vi "Initialize.vi"(8 "error in (no error)":errorcluster, 11 "Component UI in":refnum<class "Core Configuration UI.lvclass">) -> (0 "error out":errorcluster, 3 "Component UI out":refnum<class "Core Configuration UI.lvclass">)   [LabVIEW 2017, in "DSF Core.lvlib" / "Core Configuration UI.lvclass"]
uses:
  Core Configuration UI.lvclass
  C:/Git/DSF/Core/Classes/Component User Interface/Component User Interface.lvclass
  Channel/Core Channel User Interface.lvclass
  C:/Git/DSF/Core/Classes/User Interface/User Interface.lvclass
  Group/Core Group User Interface.lvclass
  Plugin/Core Plugin User Interface.lvclass
  Thread/Core Thread User Interface.lvclass
  Transfer/Core Transfer User Interface.lvclass
  Component User Interface/Component User Interface.lvclass
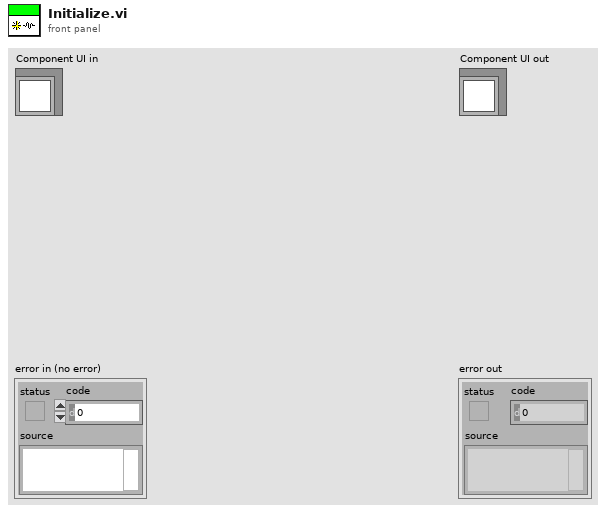
[diagram p1: front panel]
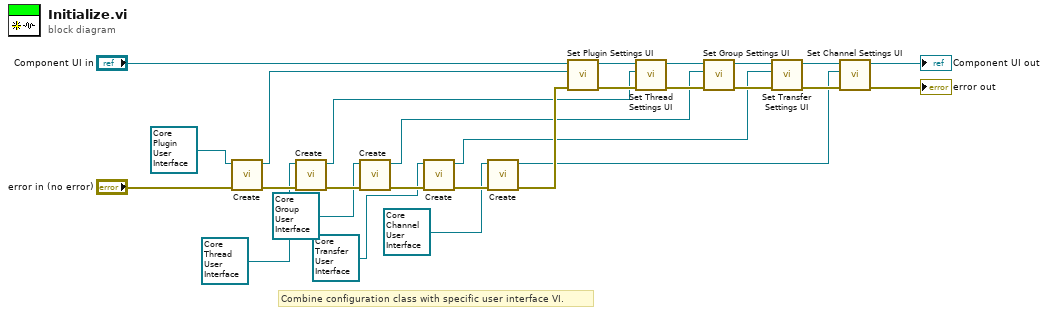
[diagram p0: block diagram]
diagram:
  # "Combine configuration class with specific user interface VI."
  n1 = call-dynamic "Create.vi"("error in (no error)"="error in (no error)", "Core Plugin User Interface in"=refnum<class "Core Plugin User Interface.lvclass"> refnum ("DSF Core.lvlib:Core Plugin User Interface.lvclass")) -> ("error out"=w5:errorcluster, "Core Plugin User Interface out"=w12:refnum<class "Core Plugin User Interface.lvclass">)  [unwired: 8 in]
  n2 = call-dynamic "Create.vi"("error in (no error)"=w5, "Core Thread User Interface in"=refnum<class "Core Thread User Interface.lvclass"> refnum ("DSF Core.lvlib:Core Thread User Interface.lvclass")) -> ("error out"=w27:errorcluster, "Core Thread User Interface out"=w11:refnum<class "Core Thread User Interface.lvclass">)  [unwired: 8 in]
  n3 = call-dynamic "Create.vi"("error in (no error)"=w27, "Core Group User Interface in"=refnum<class "Core Group User Interface.lvclass"> refnum ("DSF Core.lvlib:Core Group User Interface.lvclass")) -> ("error out"=w26:errorcluster, "Core Group User Interface out"=w10:refnum<class "Core Group User Interface.lvclass">)  [unwired: 8 in]
  n4 = call-dynamic "Create.vi"("error in (no error)"=w26, "Core Transfer User Interface in"=refnum<class "Core Transfer User Interface.lvclass"> refnum ("DSF Core.lvlib:Core Transfer User Interface.lvclass")) -> ("error out"=w25:errorcluster, "Core Transfer User Interface out"=w9:refnum<class "Core Transfer User Interface.lvclass">)  [unwired: 8 in]
  n5 = call-dynamic "Create.vi"("error in (no error)"=w25, "Core Channel User Interface in"=refnum<class "Core Channel User Interface.lvclass"> refnum ("DSF Core.lvlib:Core Channel User Interface.lvclass")) -> ("error out"=w18:errorcluster, "Core Channel User Interface out"=w8:refnum<class "Core Channel User Interface.lvclass">)  [unwired: 8 in]
  n6 = call "Set Plugin Settings UI.vi"("error in (no error)"=w18, "Plugin Settings UI"=w12, "Component UI in"="Component UI in") -> ("error out"=w17:errorcluster, "Component UI out"=w23:refnum<class "Core Configuration UI.lvclass">)  [unwired: 7 in]
  n7 = call "Set Thread Settings UI.vi"("error in (no error)"=w17, "Thread Settings UI"=w11, "Component UI in"=w23) -> ("error out"=w16:errorcluster, "Component UI out"=w22:refnum<class "Core Configuration UI.lvclass">)  [unwired: 7 in]
  n8 = call "Set Group Settings UI.vi"("error in (no error)"=w16, "Group Settings UI"=w10, "Component UI in"=w22) -> ("error out"=w15:errorcluster, "Component UI out"=w21:refnum<class "Core Configuration UI.lvclass">)  [unwired: 7 in]
  n9 = call "Set Transfer Settings UI.vi"("error in (no error)"=w15, "Transfer Settings UI"=w9, "Component UI in"=w21) -> ("error out"=w14:errorcluster, "Component UI out"=w20:refnum<class "Core Configuration UI.lvclass">)  [unwired: 7 in]
  n10 = call "Set Channel Settings UI.vi"("error in (no error)"=w14, "Channel Settings UI"=w8, "Component UI in"=w20) -> ("error out"=→"error out":errorcluster, "Component UI out"=→"Component UI out":refnum<class "Core Configuration UI.lvclass">)  [unwired: 7 in]
